vi "Launcher.vi"   [LabVIEW 2020, in "VI Properties Editor.lvlib"]
uses:
  VI Properties Editor.lvlib
types:
  T1 = enum32{"Invalid", "Standard", "Closed", "Hidden", "Minimized", "Maximized"}
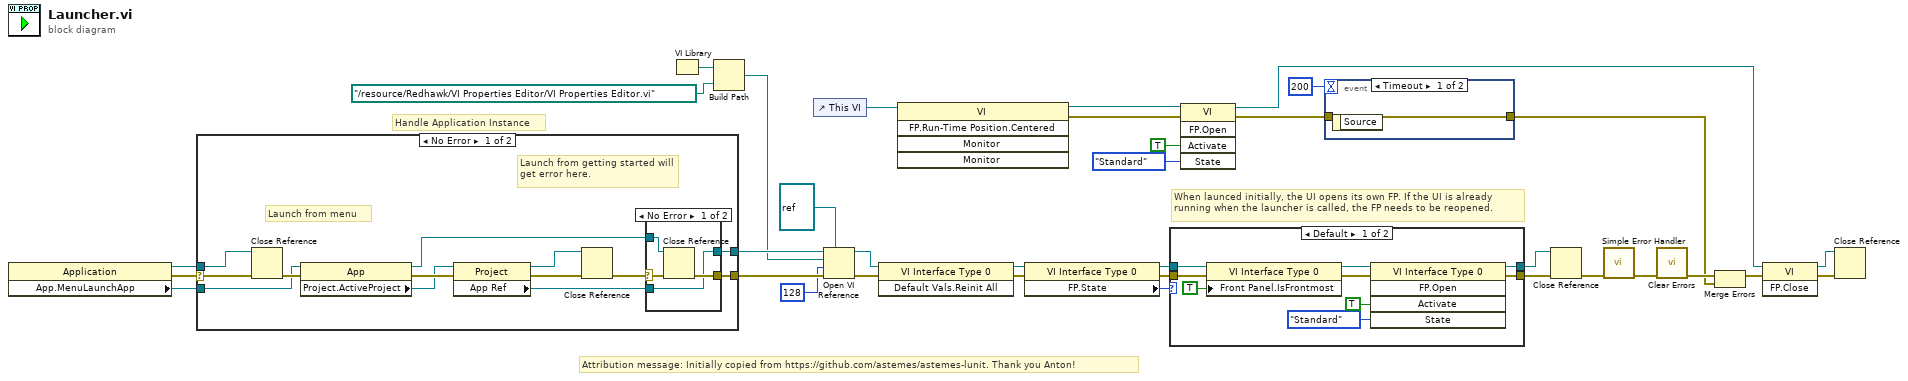
[diagram p0: block diagram]
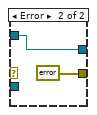
[diagram p2: hidden frame]
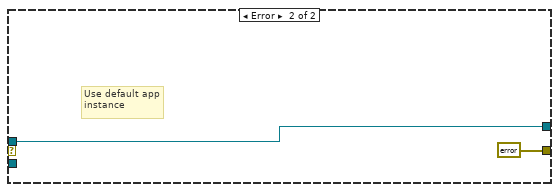
[diagram p3: hidden frame]
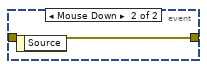
[diagram p4: hidden frame]
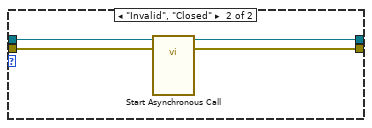
[diagram p5: hidden frame]
diagram:
  # "Attribution message: Initially copied from https://github.com/astemes/astemes-lunit. Thank you Anton!"
  # "Handle Application Instance"
  # "When launced initially, the UI opens its own FP. If the UI is already running when the launcher is called, the FP needs to be reopened."
  n1 = property class="Application"() -> (reference out=w7:refnum<vi>, error out=w22:errorcluster, "App.MenuLaunchApp"=w8:refnum<vi>)  [unwired: 2 in]
  n2 = case shown="No Error" w22 {
    selector: w22 -> [w47 _]
    tunnel: [w36 w54] -> w11
    tunnel: w8 -> [w39 _]
    tunnel: w7 -> [w41 w54]
    tunnel: [w42 errorcluster {"status"=FALSE, "code"=0, "source"=""} ("error out")] -> w24
    frame No Error {
      # "Launch from getting started will get error here."
      # "Launch from menu"
      n3 = Close Reference(reference=w41, error in (no error)=w47) -> (error out=w46:errorcluster)
      n4 = property class="App"(reference=w39, error in=w46) -> (reference out=w38:refnum<vi>, error out=w45:errorcluster, "Project.ActiveProject"=w40:refnum<vi>)
      n5 = property class="Project"(reference=w40, error in=w45) -> (reference out=w37:refnum<vi>, error out=w44:errorcluster, "App Ref"=w35:refnum<vi>)
      n6 = Close Reference(reference=w37, error in (no error)=w44) -> (error out=w43:errorcluster)
      n7 = case shown="No Error" w43 {
        selector: w43 -> [w51 _]
        tunnel: w38 -> [w49 w52]
        tunnel: [w50 errorcluster {"status"=FALSE, "code"=0, "source"=""} ("error out")] -> w42
        tunnel: [w48 w52] -> w36
        tunnel: w35 -> [w48 _]
        frame No Error {
          n8 = Close Reference(reference=w49, error in (no error)=w51) -> (error out=w50:errorcluster)
        }
        frame Error {
        }
      }
    }
    frame Error {
      # "Use default app instance"
    }
  }
  n9 = VI Library() -> (path=w3:path)
  n10 = Build Path(base path=w3, name or relative path=path "../resource/Redhawk/VI Properties Editor/VI Properties Editor.vi") -> (appended path=w9:path)
  n11 = control-ref of="This VI"() -> (w20:refnum<vi>)
  n12 = Open VI Reference(type specifier VI Refnum (for type only)=refnum<vi> refnum, application reference (local)=w11, vi path=w9, options=128, error in (no error)=w24) -> (vi reference=w10:refnum<vi>, error out=w23:errorcluster)  [unwired: 1 in]
  n13 = invoke class="VI Interface Type 0" method="Default Vals.Reinit All"(reference=w10, error in=w23) -> (reference out=w2:refnum<vi>, error out=w21:errorcluster)  [unwired: 1 in, 1 out]
  n14 = invoke class="VI" method="FP.Run-Time Position.Centered"(reference=w20) -> (reference out=w19:refnum<vi>, error out=w34:errorcluster)  [unwired: 4 in, 3 out]
  n15 = property class="VI Interface Type 0"(reference=w2, error in=w21) -> (reference out=w14:refnum<vi>, error out=w29:errorcluster, "FP.State"=w13:T1)
  n16 = case shown="Default" w13 {
    tunnel: w14 -> [w60 w66]
    tunnel: w29 -> [w64 w68]
    tunnel: [w57 w65] -> w15
    tunnel: [w62 w67] -> w33
    frame Default {
      n17 = property class="VI Interface Type 0"(reference=w60, error in=w64, "Front Panel.IsFrontmost"=TRUE ("Front Panel Window:Is Frontmost")) -> (reference out=w56:refnum<vi>, error out=w63:errorcluster)
      n18 = invoke class="VI Interface Type 0" method="FP.Open"(reference=w56, error in=w63, "Activate"=TRUE ("Activate?"), "State"=T1."Standard") -> (reference out=w57:refnum<vi>, error out=w62:errorcluster)  [unwired: 1 in, 3 out]
    }
    frame "Invalid", "Closed" {
      n19 = call-by-ref "Start Asynchronous Call"(reference=w66, error in=w68) -> (reference out=w65:refnum<vi>, error out=w67:errorcluster)  [unwired: 12 in]
    }
  }
  n20 = invoke class="VI" method="FP.Open"(reference=w19, error in=w34, "Activate"=TRUE ("Activate?"), "State"=T1."Standard") -> (reference out=w16:refnum<vi>, error out=w27:errorcluster)  [unwired: 1 in, 3 out]
  n21 = event shown="[0] Timeout" {
    selector: _ -> [_ _]
    dyn-events: _ -> [_ _]
    timeout: 200 -> [_ _]
    tunnel: w27 -> [w69 w70]
    tunnel: [w69 w70] -> w25
    event Timeout {
      n22 = event-data() -> ()  [unwired: 1 in, 1 out]
    }
    event Mouse Down {
      n23 = event-data() -> ()  [unwired: 1 in, 1 out]
    }
  }
  n24 = Close Reference(reference=w15, error in (no error)=w33) -> (error out=w31:errorcluster)
  n25 = call <vilib>:"Simple Error Handler.vi"("error in (no error)"=w31) -> ("error out"=w32:errorcluster)  [unwired: 4 in, 4 out]
  n26 = call <vilib>:"Clear Errors.vi"("error in (no error)"=w32) -> ("error out"=w30:errorcluster)  [unwired: 5 in, 1 out]
  n27 = Merge Errors(w30, w25) -> (w26:errorcluster)
  n28 = invoke class="VI" method="FP.Close"(reference=w16, error in=w26) -> (reference out=w12:refnum<vi>, error out=w28:errorcluster)  [unwired: 1 in, 1 out]
  n29 = Close Reference(reference=w12, error in (no error)=w28) -> ()  [unwired: 1 out]
